vi "Phasor Explorer Update Settings Storage.vi"(8 "Error In":errorcluster, 10 "NewVal":variant, 11 "CtlRef":refnum<vi>) -> (0 "Error Out":errorcluster)   [LabVIEW 2021, in "Phasor Explorer.lvlib"]
uses:
  Phasor Explorer.lvlib
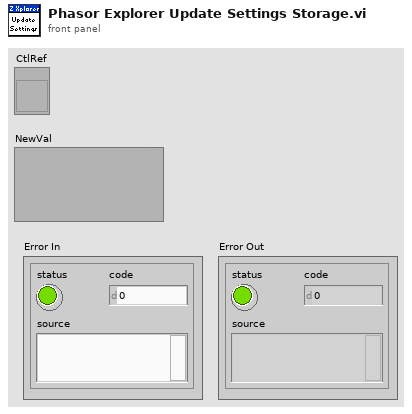
[diagram p1: front panel]
types:
  T1 = typedef "Phasor Explorer.lvlib/Phasor Explorer Settings List.ctl" = enum16{"Display Parameters", "Phasor Parameters", "Decay & IRF Parameters", "Gate Parameters", "Detector Parameters", "f*", "tau*"}
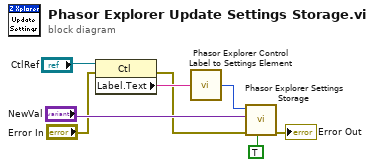
[diagram p0: block diagram]
diagram:
  n1 = property class="Ctl"(reference="CtlRef", error in="Error In") -> (error out=w2:errorcluster, "Label.Text"=w5:string)  [unwired: 1 out]
  n2 = call "Phasor Explorer Control Label to Settings Element.vi"("Label.Text"=w5) -> ("Settings List Element"=w4:T1)
  n3 = call "Phasor Explorer Settings Storage.vi"("Set/Get(F)"=TRUE, "Error In"=w2, "Variant Data in"="NewVal", "Settings List"=w4) -> ("Error Out"=→"Error Out":errorcluster)  [unwired: 6 in, 1 out]
